vi "FGV_GlobalStop.vi"(0 "Stop":bool, 4 "Enum":T1=enum."Set Soft Stop") -> (5 "Stop":bool)   [LabVIEW 2018, in "feGEM DataPacker.lvlib"]
uses:
  feGEM DataPacker.lvlib
  DataPacker_Global_Stop_Enum.ctl
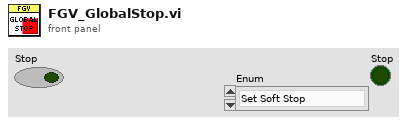
[diagram p1: front panel]
types:
  T1 = typedef "feGEM DataPacker.lvlib/DataPacker_Global_Stop_Enum.ctl" = enum16{"Reset", "Set Soft Stop", "Get Soft Stop", "Set Hard Stop", "Get Hard Stop", "Get Any Stop"}
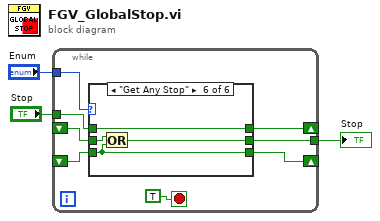
[diagram p0: block diagram]
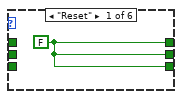
[diagram p2: hidden frame]
diagram:
  n1 = while {
    shift-right: [w10] -> _
    shift-left: _ -> [w11]
    tunnel: "Stop" -> [w8]
    tunnel: [w9] -> w1
    tunnel: "Enum" -> [w7]
    shift-right: [w5] -> _
    shift-left: _ -> [w4]
    stop <- TRUE stop-if-true
    n2 = case shown="\"Get Any Stop\"" w7 {
      tunnel: [w12 w14 w16 w17 w19 w23] -> w9
      tunnel: [w12 w14 w16 w18 w20 w22] -> w10
      tunnel: w11 -> [_ _ w16 w18 w20 w24]
      tunnel: w8 -> [_ w14 _ w17 _ w22]
      tunnel: [w12 w13 w15 w17 w19 w21] -> w5
      tunnel: w4 -> [_ w13 w15 _ w19 w21]
      frame "Reset" {
        w12 = FALSE
      }
      frame "Set Soft Stop" {
      }
      frame "Get Soft Stop", Default {
      }
      frame "Set Hard Stop" {
      }
      frame "Get Hard Stop" {
      }
      frame "Get Any Stop" {
        n3 = Or(x=w24, y=w21) -> (x .or. y?=w23:bool)
      }
    }
  }
  "Stop" <- w1
